vi "Delete Item.vi"(7 "Mode":enum16{"End", "Begin"}(ring), 8 "错误输入":errorcluster, 11 "Listbox Ref":refnum<vi>) -> (0 "错误输出":errorcluster, 3 "Dup Listbox Ref":refnum<vi>)   [LabVIEW 2011, in "Listbox Tool.lvlib"]
uses:
  Listbox Tool.lvlib
  Custom Type/Read and Write Mode.ctl
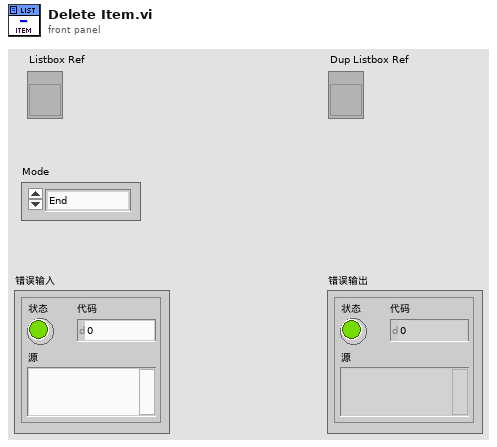
[diagram p1: front panel]
types:
  T1 = typedef "Listbox Tool.lvlib/Read and Write Mode.ctl" = enum16{"Read", "Write"}
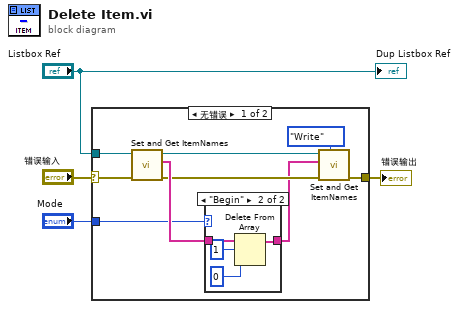
[diagram p0: block diagram]
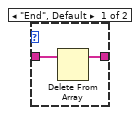
[diagram p2: hidden frame]
diagram:
  n1 = case shown="无错误" "错误输入" {
    selector: "错误输入" -> [w13 w20]
    tunnel: "Listbox Ref" -> [w12 _]
    tunnel: "Mode" -> [w7 _]
    tunnel: [w6 w20] -> w1
    frame No Error {
      n2 = call "Set and Get ItemNames.vi"("错误输入"=w13, "Listbox Ref"=w12) -> ("错误输出"=w10:errorcluster, "ItemNames Out"=w11:string[], "Dup Listbox Ref"=w9:refnum<vi>)  [unwired: 7 in]
      n3 = case shown="\"Begin\"" w7 {
        tunnel: w11 -> [w15 w19]
        tunnel: [w14 w17] -> w5
        frame "End", Default {
          n4 = Delete From Array(array=w15) -> (array with subset deleted=w14:string[])  [unwired: 2 in, 1 out]
        }
        frame "Begin" {
          n5 = Delete From Array(array=w19, length=1 ("长度"), index=0 ("索引")) -> (array with subset deleted=w17:string[])  [unwired: 1 out]
        }
      }
      n6 = call "Set and Get ItemNames.vi"("Mode"=Read_and_Write_Mode."Write", "错误输入"=w10, "ItemNames In"=w5, "Listbox Ref"=w9) -> ("错误输出"=w6:errorcluster)  [unwired: 5 in, 2 out]
    }
    frame Error {
    }
  }
  "错误输出" <- w1
  "Dup Listbox Ref" <- "Listbox Ref"
